vi "Cell Space_Excel.vi"(4 "Row Header in":string[](array[string]), 6 "Col Header in":string[](array[string]), 7 "빈내용 숨기기?(F)":bool, 8 "error in":errorcluster caption="에러 입력(에러 없음)", 10 "Data in":string[][](array[string]), 11 "report in":refnum<class "NI_report.lvclass">) -> (0 "error out":errorcluster caption="에러 출력", 1 "전체넓이":i16, 3 "report out":refnum<class "NI_report.lvclass">)   [LabVIEW 2020]
uses:
  <vilib>/Utility/NIReport.llb/NI_report.lvclass
  <vilib>/Utility/NIReport.llb/Excel/NI_Excel.lvclass
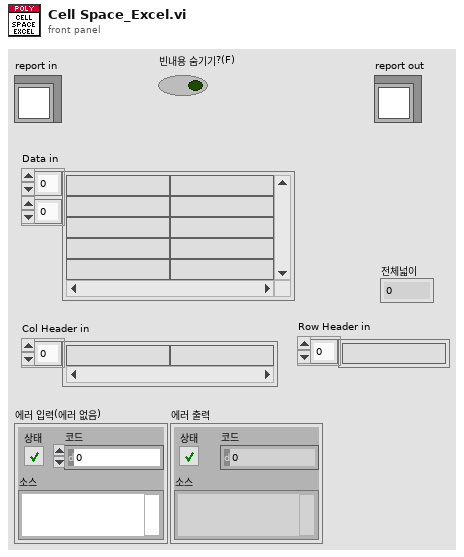
[diagram p1: front panel]
types:
  T1 = cluster{"left":i16, "top":i16, "right":i16, "bottom":i16}
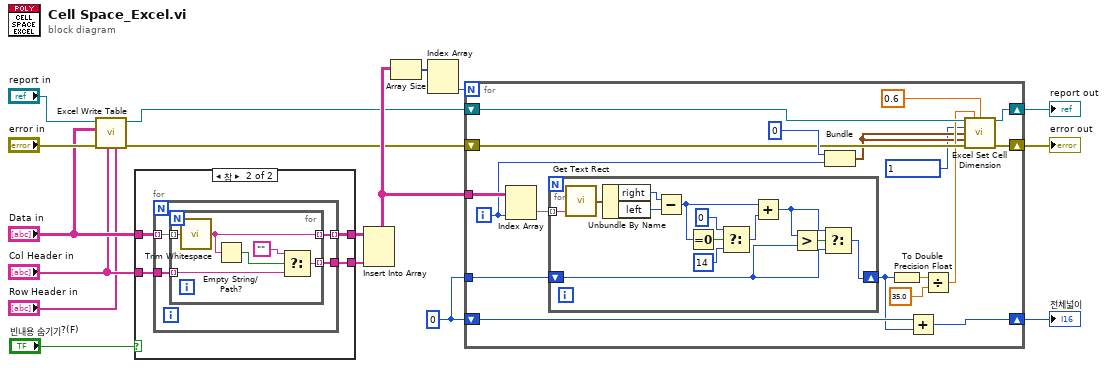
[diagram p0: block diagram]
diagram:
  w12 = i16 0 ("인덱스")
  n1 = call "Excel Write Table.vi"("행헤더"="Row Header in", "열헤더"="Col Header in", "error in"="error in", "table"="Data in", "report in"="report in") -> ("error out"=w6:errorcluster, "report out"=w4:refnum<class "NI_report.lvclass">)  [unwired: 3 in, 2 out]
  n2 = case shown="참" "빈내용 숨기기?(F)" {
    tunnel: "Data in" -> [w19 w23]
    tunnel: [w19 w22] -> w9
    tunnel: "Col Header in" -> [w18 w21]
    tunnel: [w18 w20] -> w8
    frame False {
    }
    frame True {
      n3 = for {
        tunnel: w23 -> [w27] mode=indexing
        tunnel: [w26] -> w22 mode=indexing
        tunnel: w21 -> [w25]
        tunnel: [w24] -> w20
        n4 = for {
          tunnel: w27 -> [w33] mode=indexing
          tunnel: [w32] -> w26 mode=indexing
          tunnel: w25 -> [w30] mode=indexing
          tunnel: [w29] -> w24 mode=indexing
          n5 = call <vilib>:"Trim Whitespace.vi"("string"=w33) -> ("trimmed string"=w32:string)  [unwired: 1 in]
          n6 = Empty String/Path?(string/path=w32) -> (empty?=w31:bool)
          n7 = Select(t="", s=w31, f=w30) -> (s? t:f=w29:string)
        }
      }
    }
  }
  n8 = Insert Into Array(array=w9, new element=w8) -> (w11:string[][])  [unwired: 2 in]
  n9 = Array Size(array=w11) -> (size(s)=w17:i32[])
  n10 = Index Array(array=w17) -> (element #2=w16:i32)  [unwired: 2 in, 1 out]
  n11 = for {
    N: w16 -> [_]
    shift-right: [w45] -> w15
    shift-left: w6 -> [w44]
    tunnel: w11 -> [w51]
    shift-right: [w47] -> w14
    shift-left: w12 -> [w46]
    shift-right: [w42] -> w13
    shift-left: w4 -> [w43]
    tunnel: w12 -> [w34]
    i -> [w49]
    n12 = Index Array(array=w51, index (col)=w49) -> (element=w50:string[])  [unwired: 1 in]
    n13 = for {
      tunnel: w50 -> [w61] mode=indexing
      shift-right: [w62] -> w40
      shift-left: w34 -> [w63]
      n14 = call <vilib>:"Get Text Rect.vi"("text"=w61) -> ("rect"=w60:T1)  [unwired: 8 in]
      n15 = Unbundle By Name(w60) -> ("right"=w59:i16, "left"=w58:i16)
      n16 = Subtract(x=w59, y=w58) -> (x-y=w56:i16)
      n17 = Equal To 0?(x=w56) -> (x = 0?=w55:bool)
      n18 = Select(t=i16 0 ("y"), s=w55, f=i16 14 ("y")) -> (s? t:f=w52:i16)
      n19 = Add(x=w56, y=w52) -> (x+y=w57:i16)
      n20 = Greater?(x=w57, y=w63) -> (0:w64:bool)
      n21 = Select(t=w57, s=w64, f=w63) -> (s? t:f=w62:i16)
    }
    n22 = Bundle("인덱스"=0, w49) -> (w36:cluster{"인덱스":i32, i32})  [unwired: 1 in]
    n23 = To Double Precision Float(number=w40) -> (double precision float=w39:dbl)
    n24 = Add(x=w46, y=w40) -> (x+y=w47:i16)
    n25 = Divide(x=w39, y=35.0) -> (x/y=w37:dbl)
    n26 = call <vilib>:"Excel Set Cell Dimension.vi"("report in"=w43, "width (-1)"=w37, "height (-1)"=0.6, "measurement system"=u16 1, "start (-1, -1)"=w36, "end (-1, -1)"=w36, "error in (no error)"=w44) -> ("report out"=w42:refnum<class "NI_report.lvclass">, "error out"=w45:errorcluster)  [unwired: 7 in]
  }
  "error out" <- w15
  "전체넓이" <- w14
  "report out" <- w13
